vi "Find Class in Memory Test.vi"() -> (2 "Result":bool)   [LabVIEW 2014, in "SystemConfigReop Tests.lvlib"]
uses:
  SystemConfigReop Tests.lvlib
  Configuration Editor/Classes/Systems/Systems.lvclass
  Configuration Editor/Classes/Targets/Targets.lvclass
  Configuration Editor/Classes/SystemConfigRepo/SystemConfigRepo.lvclass
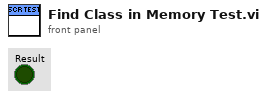
[diagram p1: front panel]
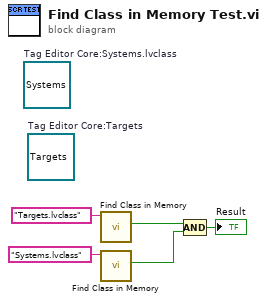
[diagram p0: block diagram]
diagram:
  (unwired) refnum<class "Targets.lvclass"> refnum  # Tag Editor Core:Targets
  (unwired) refnum<class "Systems.lvclass"> refnum  # Tag Editor Core:Systems.lvclass
  n1 = call "Find Class in Memory.vi"("Class Name"="Targets.lvclass") -> ("Class Found?"=w3:bool)  [unwired: 9 in, 1 out]
  n2 = call "Find Class in Memory.vi"("Class Name"="Systems.lvclass") -> ("Class Found?"=w2:bool)  [unwired: 9 in, 1 out]
  n3 = Compound Arithmetic op=AND(w3, w2) -> (→"Result":bool)
